vi "PBcard_both_close.vi"(0 "error in (no error)":errorcluster) -> (2 "error out":errorcluster)   [LabVIEW 2013, in "PulseBlaster.lvlib"]
doc: "This vi sends a software trigger to the PulseBlaster.\n\nIn order to start the PulseBlaster, the following sequence must occur, even if the PulseBlaster is not reprogrammed, but merely retriggered:\n1) Reset the PulseBlaster\n2) Load number of bytes per word\n3) Select Memory device (external or internal)\n4) Clear address counter\n5) Send program finished\n6) Send the \"start\" trigger.\n\nThe inputs should rarely be changed, as they are hardware specific."
uses:
  PulseBlaster.lvlib
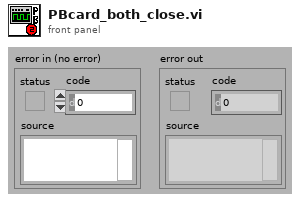
[diagram p1: front panel]
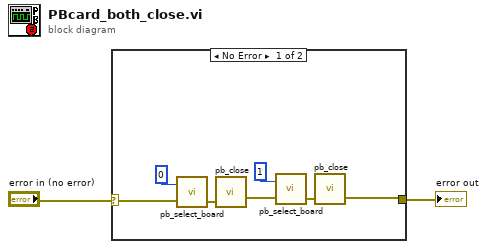
[diagram p0: block diagram]
diagram:
  n1 = case shown="No Error" "error in (no error)" {
    selector: "error in (no error)" -> [w8 w10]
    tunnel: [w3 w10] -> w1
    frame No Error {
      n2 = call "pb_select_board.vi"("error in (no error)"=w8, "Board to Address"=0) -> ("error out"=w9:errorcluster)
      n3 = call "pb_close.vi"("error in (no error)"=w9) -> ("error out"=w4:errorcluster)
      n4 = call "pb_select_board.vi"("error in (no error)"=w4, "Board to Address"=1) -> ("error out"=w6:errorcluster)
      n5 = call "pb_close.vi"("error in (no error)"=w6) -> ("error out"=w3:errorcluster)
    }
    frame Error {
    }
  }
  "error out" <- w1
